vi "Cam change inner param.vi"(8 "error in (no error)":errorcluster, 11 "Camera in":refnum<class "Camera.lvclass">) -> (0 "error out":errorcluster, 3 "Camera out":refnum<class "Camera.lvclass">)   [LabVIEW 2021, in "Camera.lvlib" / "Camera.lvclass"]
uses:
  Camera.lvclass
  Camera.lvclass/Camera.ctl
panel:
  in  "OK Button":bool
  in  "Cam inner parameters":T1
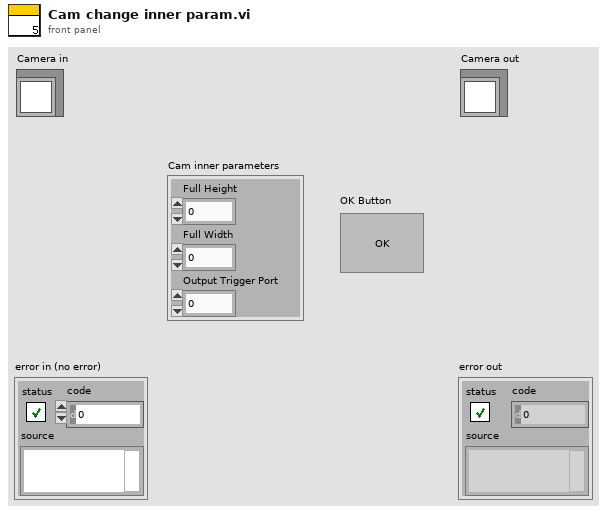
[diagram p1: front panel]
types:
  T1 = cluster{"Full Height":dbl, "Full Width":dbl, "Output Trigger Port":dbl}
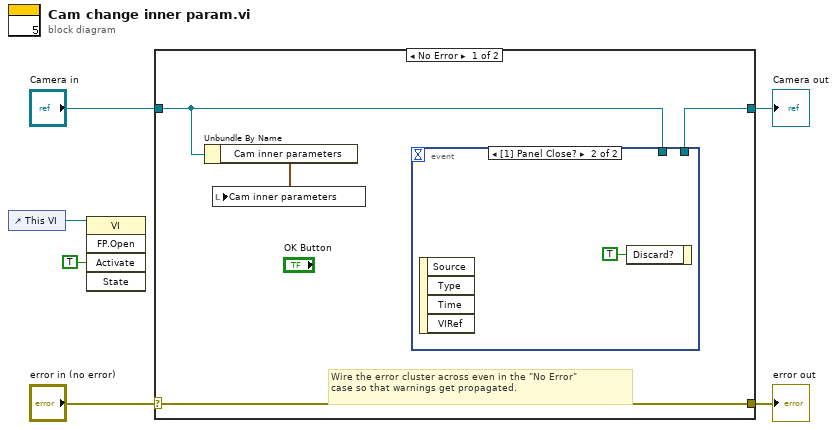
[diagram p0: block diagram]
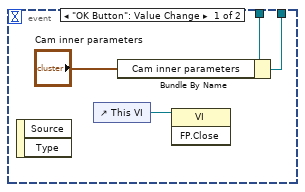
[diagram p2: hidden frame]
diagram:
  n1 = control-ref of="This VI"() -> (w2:refnum<vi>)
  n2 = invoke class="VI" method="FP.Open"(reference=w2, "Activate"=TRUE ("Activate?")) -> ()  [unwired: 3 in, 5 out]
  n3 = case shown="No Error" "error in (no error)" {
    selector: "error in (no error)" -> [w10 w17]
    tunnel: [w10 w17] -> w5
    tunnel: [w7 w16] -> w3
    tunnel: "Camera in" -> [w8 w16]
    frame No Error {
      # "Wire the error cluster across even in the \"No Error\"\ncase so that warnings get propagated."
      n4 = Unbundle By Name(w8) -> ("Cam inner parameters"=w9:T1)
      n5 = local write "Cam inner parameters"(w9) -> ()
      n6 = event shown="[1] Panel Close?" {
        selector: _ -> [_ _]
        dyn-events: _ -> [_ _]
        timeout: _ -> [_ _]
        tunnel: w8 -> [w14 _]
        tunnel: [w11 _] -> w7
        event "OK Button": Value Change {
          n7 = event-data() -> ()  [unwired: 1 in, 2 out]
          n8 = control-ref of="This VI"() -> (w12:refnum<vi>)
          n9 = Bundle By Name(cluster=w14, "Cam inner parameters"="Cam inner parameters") -> (w11:refnum<class "Camera.lvclass">)
          n10 = invoke class="VI" method="FP.Close"(reference=w12) -> ()  [unwired: 2 in, 3 out]
        }
        event Panel Close? {
          n11 = event-data() -> ()  [unwired: 1 in, 4 out]
          n12 = event-data("Discard?"=TRUE) -> ()  [unwired: 1 in, 1 out]
        }
      }
    }
    frame Error {
    }
  }
  "error out" <- w5
  "Camera out" <- w3
